vi "Mosfet_Modified.vi"() -> ()   [LabVIEW 2013]
uses:
  <vilib>/Instr/_visa.llb/VISA Event Mechanism.ctl
  <vilib>/Instr/_visa.llb/Select Event Type.ctl
panel:
  out "XY Graph":cluster{dbl[], dbl[]}(graph)
  out "Current (A)   Voltage (V)":dbl[][](array[numeric])
  out "error out":errorcluster={"status"=TRUE, "code"=-1073807346, "source"="VISA Open in 4200MOSFETexample1.vi"}
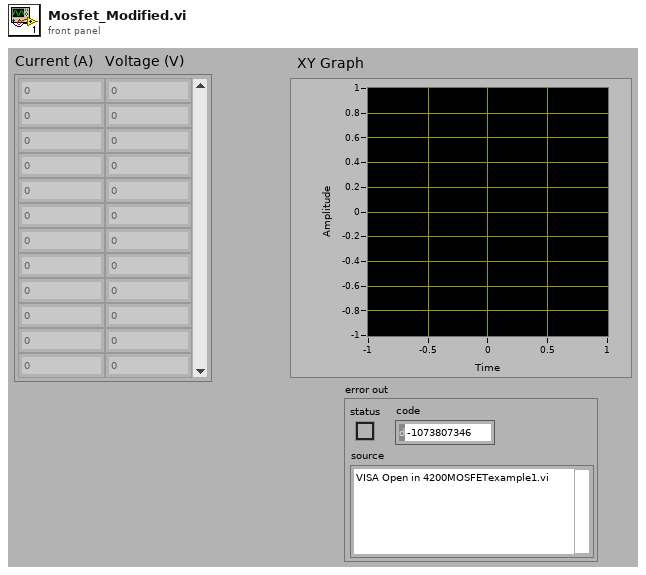
[diagram p1: front panel]
types:
  T1 = typedef "Select Event Type.ctl" = u32
  T2 = typedef "VISA Event Mechanism.ctl" = u16
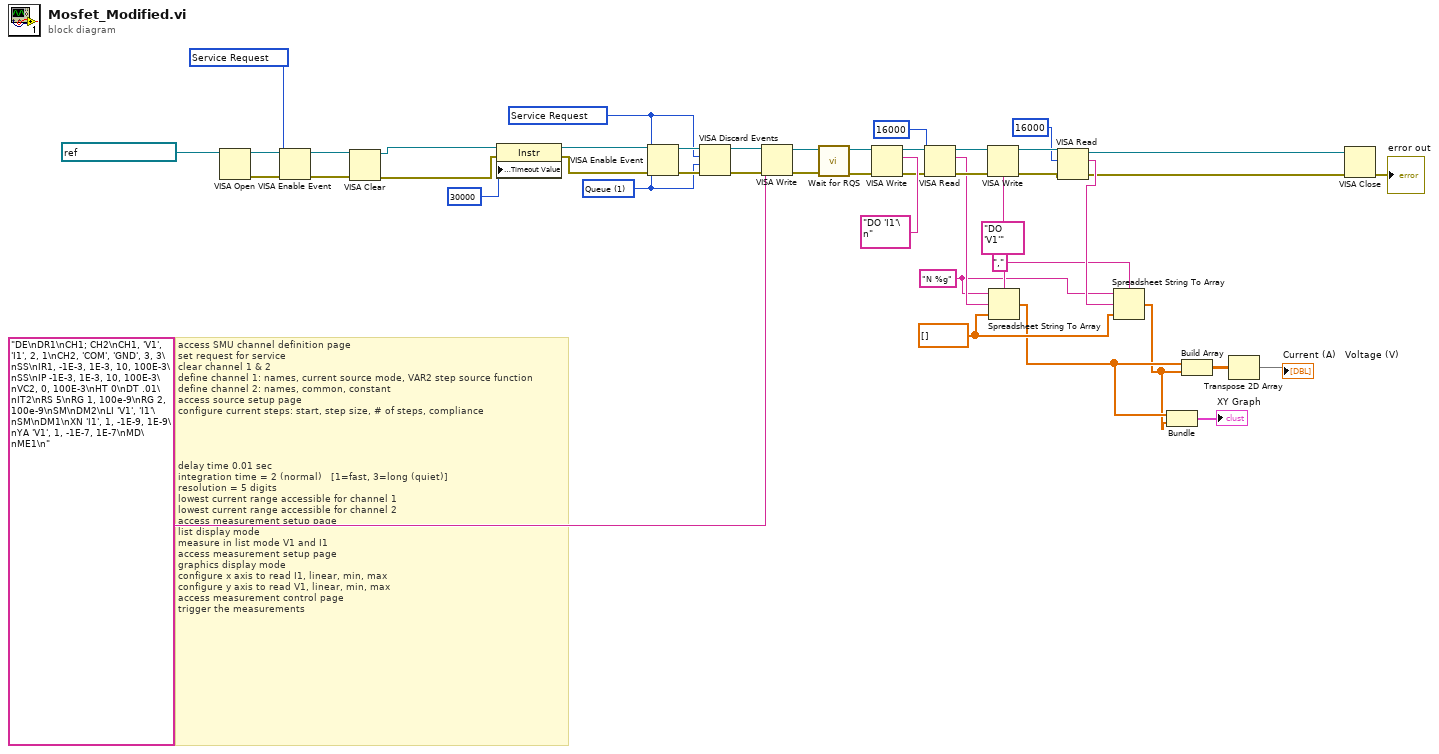
[diagram p0: block diagram]
diagram:
  w28 = T1 1073684491 items=["Service Request"=1073684491, "Trigger"=3221168138, "Clear"=1073684493, "VXI Signal"=1073684512, "VXI/VME Interrupt"=3221168161, "VXI/VME Sysfail"=1073684509, "VXI/VME Sysreset"=1073684510, "GPIB CIC"=1073684498, "GPIB Talk"=1073684499, "GPIB Listen"=1073684500, "PXI Interrupt"=1073684514, "Serial Break"=1073684515, "Serial TermChar"=1073684516, "Serial CTS"=1073684521, "Serial DSR"=1073684522, "Serial DCD"=1073684524, "Serial RI"=1073684526, "Serial Character"=1073684533, "USB Interrupt"=1073684535, "All Enabled"=1073709055] ("Event Type")
  w9 = dbl[] []
  w11 = "," ("delimiter (Tab)")
  w10 = "N %g" ("format string")
  w39 = T2 1 items=["Queue"=1] ("Mechanism Type")
  w40 = T1 1073684491 items=["Service Request"=1073684491, "Trigger"=3221168138, "Clear"=1073684493, "VXI Signal"=1073684512, "VXI/VME Interrupt"=3221168161, "VXI/VME Sysfail"=1073684509, "VXI/VME Sysreset"=1073684510, "GPIB CIC"=1073684498, "GPIB Talk"=1073684499, "GPIB Listen"=1073684500, "PXI Interrupt"=1073684514, "Serial Break"=1073684515, "Serial TermChar"=1073684516, "Serial CTS"=1073684521, "Serial DSR"=1073684522, "Serial DCD"=1073684524, "Serial RI"=1073684526, "Serial Character"=1073684533, "USB Interrupt"=1073684535, "All Enabled"=1073709055] ("Event Type")
  # "access SMU channel definition page\nset request for service\nclear channel 1 & 2\ndefine channel 1: names, current source mode, VAR2 step source function\ndefine channel 2: names, common, constant\naccess source setup page\nconfigure current steps: start, step size, # of steps, compliance\n\n\n\n\ndelay time 0.01 sec\nintegration time = 2 (normal)   [1=fast, 3=long (quiet)]\nresolution = 5 digits\nlowest current range accessible for channel 1\nlowest current range accessible for channel 2\naccess measurement setup page\nlist display mode\nmeasure in list mode V1 and I1\naccess measurement setup page\ngraphics display mode\nconfigure x axis to read I1, linear, min, max\nconfigure y axis to read V1, linear, min, max\naccess measurement control page\ntrigger the measurements"
  n1 = VISA Open(VISA resource name=refnum<visa-resource-name> "GPIB0::17::INSTR") -> (VISA resource name=w31:refnum<visa-resource-name>, error out=w32:errorcluster)  [unwired: 1 in, 3 out]
  n2 = VISA Enable Event(8:w32, 10:w28, 11:w31) -> (0:w29:errorcluster, 3:w30:refnum<visa-resource-name>)  [unwired: 1 out]
  n3 = VISA Clear(VISA resource name=w30, error in (no error)=w29) -> (VISA resource name out=w38:refnum<visa-resource-name>, error out=w37:errorcluster)
  n4 = property class="Instr"(reference=w38, error in=w37, "General Settings:Timeout Value"=u32 30000) -> (reference out=w36:refnum<visa-resource-name>, error out=w35:errorcluster)
  n5 = VISA Enable Event(8:w35, 9:w39, 10:w40, 11:w36) -> (0:w41:errorcluster, 3:w42:refnum<visa-resource-name>)
  n6 = VISA Discard Events(8:w41, 9:w39, 10:w40, 11:w42) -> (0:w34:errorcluster, 3:w33:refnum<visa-resource-name>)
  n7 = VISA Write(VISA resource name=w33, write buffer="DE\nDR1\nCH1; CH2\nCH1, 'V1', 'I1', 2, 1\nCH2, 'COM', 'GND', 3, 3\nSS\nIR1, -1E-3, 1E-3, 10, 100E-3\nSS\nIP -1E-3, 1E-3, 10, 100E-3\nVC2, 0, 100E-3\nHT 0\nDT .01\nIT2\nRS 5\nRG 1, 100e-9\nRG 2, 100e-9\nSM\nDM2\nLI 'V1', 'I1'\nSM\nDM1\nXN 'I1', 1, -1E-9, 1E-9\nYA 'V1', 1, -1E-7, 1E-7\nMD\nME1\n", error in (no error)=w34) -> (VISA resource name out=w27:refnum<visa-resource-name>, error out=w26:errorcluster)  [unwired: 1 out]
  n8 = call <vilib>:"Wait for RQS.vi"("error in (no error)"=w26, "VISA resource name"=w27) -> ("error out"=w23:errorcluster, "VISA resource name out"=w25:refnum<visa-resource-name>)  [unwired: 1 in, 7 out]
  n9 = VISA Write(VISA resource name=w25, write buffer="DO 'I1'\n", error in (no error)=w23) -> (VISA resource name out=w24:refnum<visa-resource-name>, error out=w19:errorcluster)  [unwired: 1 out]
  n10 = VISA Read(VISA resource name=w24, byte count=u32 16000, error in (no error)=w19) -> (VISA resource name out=w21:refnum<visa-resource-name>, read buffer=w13:string, error out=w17:errorcluster)  [unwired: 1 out]
  n11 = VISA Write(VISA resource name=w21, write buffer="DO 'V1'", error in (no error)=w17) -> (VISA resource name out=w15:refnum<visa-resource-name>, error out=w16:errorcluster)  [unwired: 1 out]
  n12 = Spreadsheet String To Array(delimiter (Tab)=w11, format string=w10, spreadsheet string=w13, array type (2D Dbl)=w9) -> (array=w5:dbl[])
  n13 = VISA Read(VISA resource name=w15, byte count=u32 16000, error in (no error)=w16) -> (VISA resource name out=w7:refnum<visa-resource-name>, read buffer=w12:string, error out=w6:errorcluster)  [unwired: 1 out]
  n14 = Spreadsheet String To Array(delimiter (Tab)=w11, format string=w10, spreadsheet string=w12, array type (2D Dbl)=w9) -> (array=w4:dbl[])
  n15 = Bundle(w5, w4) -> (→"XY Graph":cluster{dbl[], dbl[]})  [unwired: 1 in]
  n16 = Build Array(w5, w4) -> (w2:dbl[][])
  n17 = Transpose 2D Array(2D array=w2) -> (transposed array=→"Current (A)   Voltage (V)":dbl[][])
  n18 = VISA Close(VISA resource name=w7, error in (no error)=w6) -> (error out=→"error out":errorcluster)
